vi "Read_Barcode_STN10.vi"(5 "Enum":T2=enum."Close", 6 "error in (no error)":errorcluster, 7 "Serial Settings":T1={"Com Port Number"="COM21", "Baud Rate"=9600, "Data Bits"=8, "Parity"=enum."None", "Stop Bits"=10, "Flow Control"=0} {"Baud Rate" items=["75"=75, "110"=110, "134"=134, "150"=150, "300"=300, "600"=600, "1200"=1200, "1800"=1800, "2400"=2400, "4800"=4800, "7200"=7200, "9600"=9600, "14400"=14400, "19200"=19200, "28800"=28800, "38400"=38400, "56000"=56000, "57600"=57600, "115200"=115200, "128000"=128000, "230400"=230400]; "Stop Bits" items=["1.0"=10, "1.5"=15, "2.0"=20]; "Flow Control" items=["None"=0, "XON/XOFF"=1, "RTS/CTS"=2, "DTR/DSR"=4]}, 9 "Visa In":refnum<visa-resource-name>="COM24") -> (0 "error out":errorcluster, 2 "Buffer Out":string, 3 "VISA Out":refnum<visa-resource-name>, 4 "Read":bool)   [LabVIEW 2020]
uses:
  Controls/Action Enum.ctl
  Controls/Com_Settings.ctl
  <vilib>/Instr/_visa.llb/VISA Configure Serial Port (Instr).vi
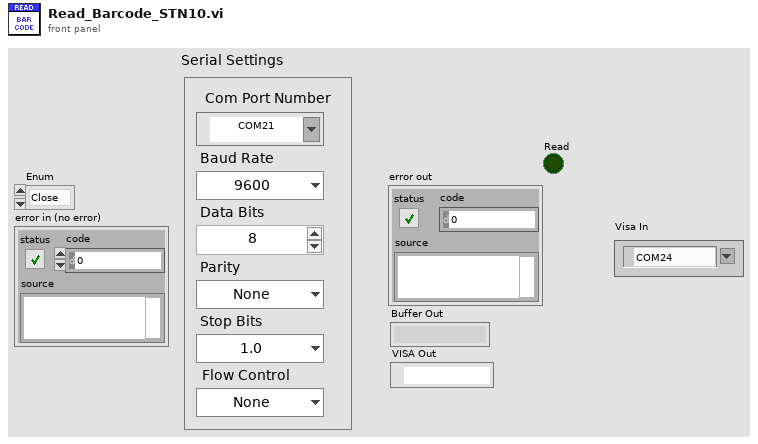
[diagram p1: front panel]
types:
  T1 = typedef "Com_Settings.ctl" = cluster{"Com Port Number":refnum<visa-resource-name>, "Baud Rate":u32, "Data Bits":u16, "Parity":enum16{"None", "Odd", "Even", "Mark", "Space"}, "Stop Bits":u16, "Flow Control":u16}
  T2 = typedef "Action Enum.ctl" = enum16{"Open", "Read", "Write", "Close"}
  T3 = cluster{"baud rate":u32, "data bits":u16, "parity":enum16{"None", "Odd", "Even", "Mark", "Space"}, "stop bits":u16, "flow control":u16}
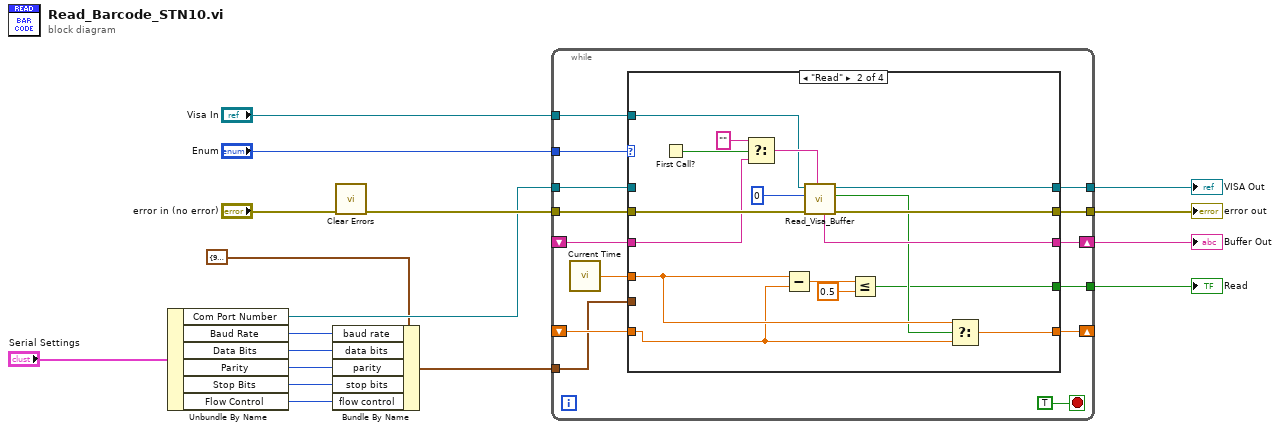
[diagram p0: block diagram]
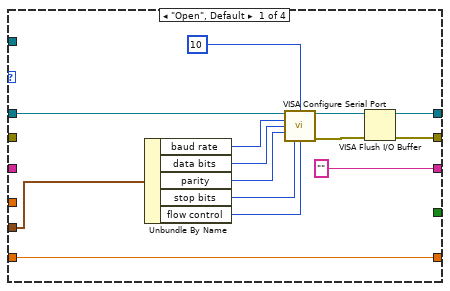
[diagram p2: hidden frame]
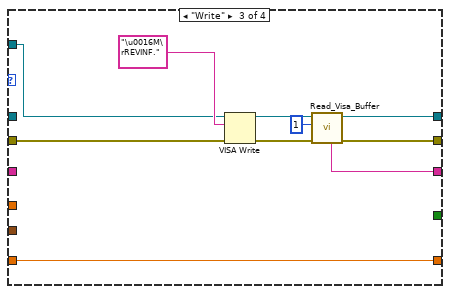
[diagram p3: hidden frame]
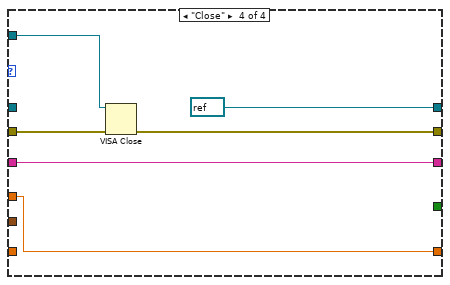
[diagram p4: hidden frame]
diagram:
  n1 = Unbundle By Name("Serial Settings") -> ("Com Port Number"=w8:refnum<visa-resource-name>, "Baud Rate"=w6:u32, "Data Bits"=w5:u16, "Parity"=w4:enum16{"None", "Odd", "Even", "Mark", "Space"}, "Stop Bits"=w3:u16, "Flow Control"=w2:u16)
  n2 = Bundle By Name(cluster=T3 {"baud rate"=9600, "data bits"=8, "parity"=enum."None", "stop bits"=10, "flow control"=0} ("Serial Settings"), "baud rate"=w6, "data bits"=w5, "parity"=w4, "stop bits"=w3, "flow control"=w2) -> (w1:T3)
  n3 = call <vilib>:"Clear Errors.vi"("error in (no error)"="error in (no error)") -> ("error out"=w12:errorcluster)  [unwired: 5 in, 1 out]
  n4 = while {
    tunnel: "Visa In" -> [w31]
    tunnel: "Enum" -> [w27]
    shift-right: [w26] -> w13
    shift-left: _ -> [w25]
    tunnel: [w24] -> w15
    tunnel: w12 -> [w23]
    tunnel: [w22] -> w11
    shift-right: [w20] -> _
    shift-left: _ -> [w19]
    tunnel: w8 -> [w28]
    tunnel: [w29] -> w10
    tunnel: w1 -> [w18]
    stop <- TRUE stop-if-true
    n5 = call <userlib>:"Current Time.vi"() -> ("Current Time (Sec)"=w21:dbl)  [unwired: 15 in]
    n6 = case shown="\"Read\"" w27 {
      tunnel: w31 -> [_ w48 w69 w73]
      tunnel: [w35 w61 w65 refnum<visa-resource-name> refnum ("VISA Refnum out")] -> w29
      tunnel: w28 -> [w32 _ _ _]
      tunnel: ["" ("Buffer Out") w60 w64 w75] -> w26
      tunnel: w25 -> [_ w51 _ w75]
      tunnel: [w34 w58 w66 w77] -> w24
      tunnel: w23 -> [_ w59 w71 w78]
      tunnel: [_ w46 _ _] -> w22
      tunnel: w21 -> [_ w56 _ w74]
      tunnel: [w38 w57 w70 w74] -> w20
      tunnel: w19 -> [w38 w55 w70 _]
      tunnel: w18 -> [w33 _ _ _]
      frame "Open", Default {
        n7 = Unbundle By Name(w33) -> ("baud rate"=w45:u32, "data bits"=w44:u16, "parity"=w43:enum16{"None", "Odd", "Even", "Mark", "Space"}, "stop bits"=w42:u16, "flow control"=w41:u16)
        n8 = call-poly "VISA Configure Serial Port"("VISA resource name"=w32, "termination char\n(0xA = '\\n' = LF)"=u8 10 ("termination char\n(0xA = '\\n' = LF)"), "baud rate (9600)"=w45, "data bits (8)"=w44, "parity (0:none)"=w43, "stop bits (10: 1 bit)"=w42, "flow control (0:none)"=w41) -> ("VISA resource name out"=w37:refnum<visa-resource-name>, "error out"=w36:errorcluster)  [unwired: 3 in, 4 out]
        n9 = VISA Flush I/O Buffer(VISA resource name=w37, error in (no error)=w36) -> (VISA resource name out=w35:refnum<visa-resource-name>, error out=w34:errorcluster)  [unwired: 1 in]
      }
      frame "Read" {
        n10 = First Call?() -> (First Call?: T/F=w52:bool)
        n11 = Select(t="", s=w52, f=w51) -> (s? t:f=w49:string)
        n12 = Subtract(x=w56, y=w55) -> (x-y=w54:dbl)
        n13 = call "Read_Visa_Buffer.vi"("Buffer In"=w49, "error in (no error)"=w59, "delay before read (ms)"=u32 0, "VISA Refnum in"=w48) -> ("error out"=w58:errorcluster, "Read"=w47:bool, "VISA Refnum out"=w61:refnum<visa-resource-name>, "Buffer Out"=w60:string)  [unwired: 2 in]
        n14 = Less Or Equal?(x=w54, y=0.5) -> (x <= y?=w46:bool)
        n15 = Select(t=w56, s=w47, f=w55) -> (s? t:f=w57:dbl)
      }
      frame "Write" {
        n16 = VISA Write(VISA resource name=w69, write buffer="\u0016M\rREVINF.", error in (no error)=w71) -> (VISA resource name out=w68:refnum<visa-resource-name>, error out=w67:errorcluster)  [unwired: 1 out]
        n17 = call "Read_Visa_Buffer.vi"("error in (no error)"=w67, "delay before read (ms)"=u32 1, "VISA Refnum in"=w68) -> ("error out"=w66:errorcluster, "VISA Refnum out"=w65:refnum<visa-resource-name>, "Buffer Out"=w64:string)  [unwired: 3 in, 1 out]
      }
      frame "Close" {
        n18 = VISA Close(VISA resource name=w73, error in (no error)=w78) -> (error out=w77:errorcluster)
      }
    }
  }
  "error out" <- w15
  "Buffer Out" <- w13
  "Read" <- w11
  "VISA Out" <- w10
